vi "G#Object_UnregisterObject.vi"(0 "reference in":refnum<class "G#Object.lvclass">, 1 "object information":T1, 2 "object killed":bool, 3 "forced destroy":bool, 5 "error in (no error)":errorcluster) -> (14 "reference out":refnum<class "G#Object.lvclass">, 19 "error out":errorcluster)   [LabVIEW 2020, in "G#Object.lvclass"]
doc: "Unregisters the object from the G# object lists. It also sends an event to the debugger and desktop trace."
uses:
  <vilib>/addons/_AddQ/G#Object/G#Object.lvclass
  <vilib>/addons/_AddQ/G#Object/utils/G#Object_ObjectInfoType.ctl
  <vilib>/addons/_AddQ/G#Object/utils/G#Object_CreateMethod.ctl
  <vilib>/addons/_AddQ/G#Object/G#Object.lvclass/G#Object.ctl
  <vilib>/addons/_AddQ/G#Object/utils/G#Object_EventType.ctl
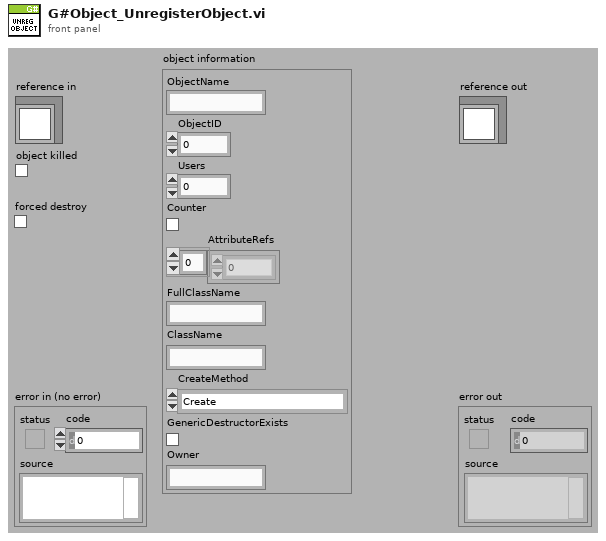
[diagram p1: front panel]
types:
  T1 = typedef "G#Object.lvclass/G#Object_ObjectInfoType.ctl" = cluster{"ObjectName":string, "ObjectID":u32, "Users":i32, "Counter":bool, "AttributeRefs":u32[], "FullClassName":string, "ClassName":string, "CreateMethod":T2, "GenericDestructorExists":bool, "Owner":string}
  T2 = typedef "G#Object.lvclass/G#Object_CreateMethod.ctl" = enum16{"Create", "Create or look up existing", "Look up existing"}
  T3 = typedef "G#Object.lvclass/G#Object_EventType.ctl" = enum16{"Created new", "Looked up existing", "Deleted", "Forced delete", "Not deleted", "Garbage collected", "Cleared", "User", "Error", "External create object", "External create class attributes", "Created class attributes", "Run constructor", "Run constructor done", "Run open method", "Run open method done"}
  T4 = cluster{"full class name (\"\")":string, "Ref":refnum<class "G#Object.lvclass">}
  T5 = cluster{"full class name (\"\")":string, "Ref":refnum<class "G#Object.lvclass">}[]
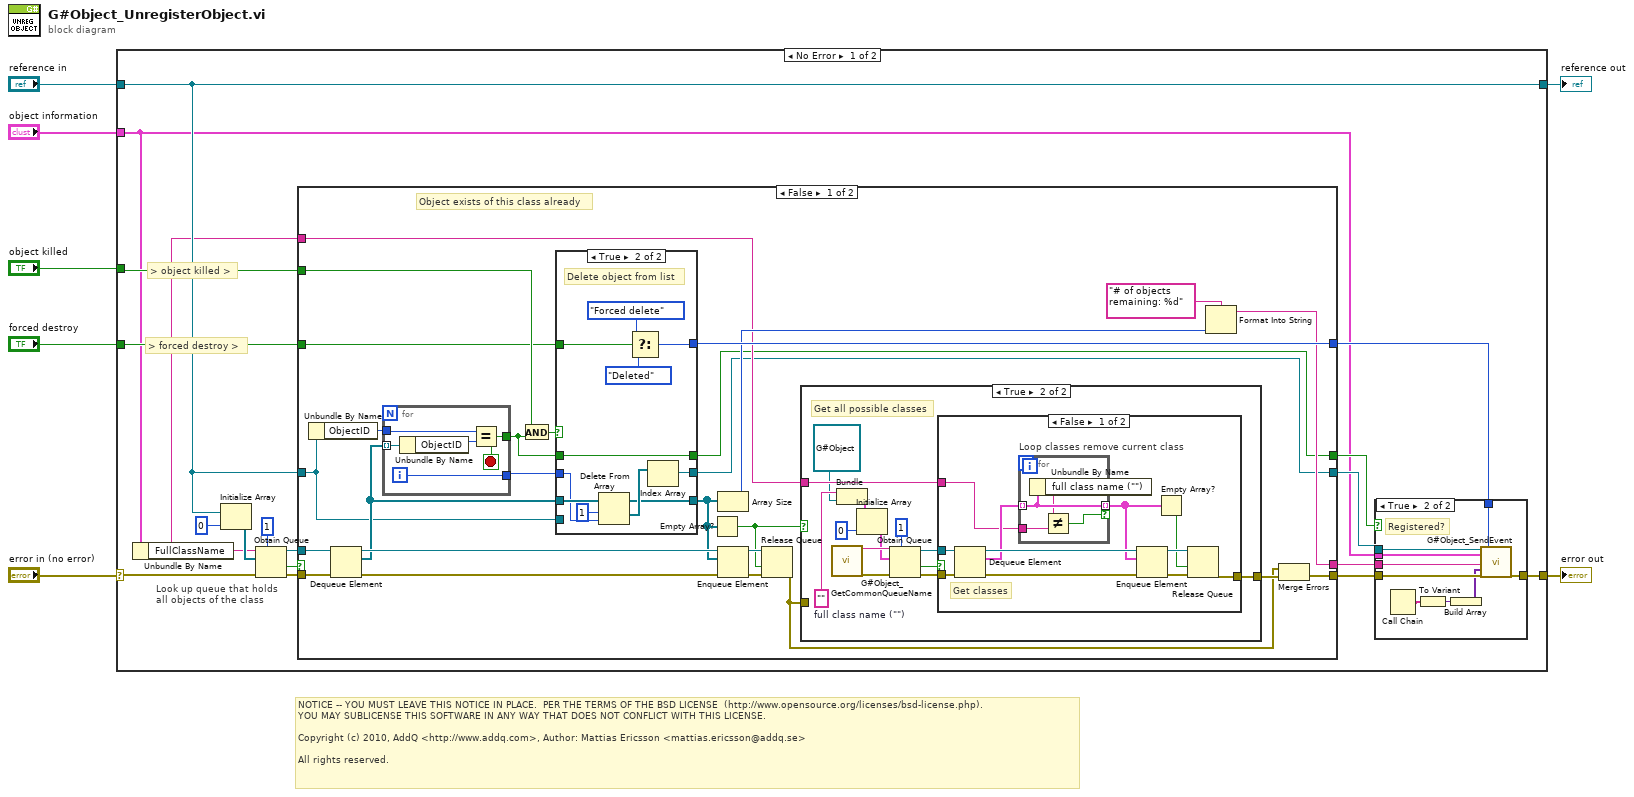
[diagram p0: block diagram]
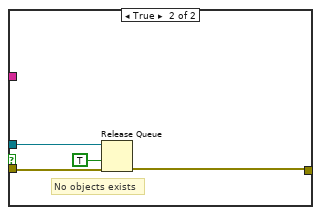
[diagram p4: hidden frame]
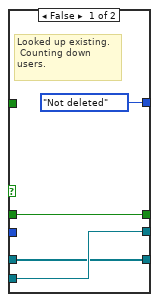
[diagram p5: hidden frame]
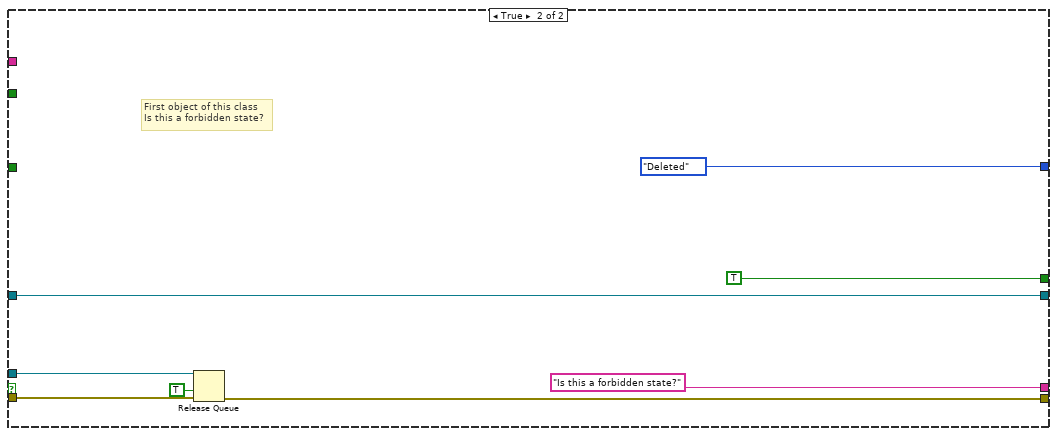
[diagram p6: hidden frame]
diagram:
  # "NOTICE -- YOU MUST LEAVE THIS NOTICE IN PLACE.  PER THE TERMS OF THE BSD LICENSE  (http://www.opensource.org/licenses/bsd-license.php).\nYOU MAY SUBLICENSE THIS SOFTWARE IN ANY WAY THAT DOES NOT CONFLICT WITH THIS LICENSE.\n\nCopyright (c) 2010, AddQ <http://www.addq.com>, Author: Mattias Ericsson <mattias.ericsson@addq.se>\n\nAll rights reserved."
  n1 = case shown="No Error" "error in (no error)" {
    selector: "error in (no error)" -> [w15 w123]
    tunnel: [w16 w123] -> w6
    tunnel: [w14 w122] -> w4
    tunnel: "reference in" -> [w14 w122]
    tunnel: "object killed" -> [w18 _]
    tunnel: "forced destroy" -> [w17 _]
    tunnel: "object information" -> [w9 _]
    frame No Error {
      # "> object killed >"
      # "> forced destroy >"
      # "Look up queue that holds\nall objects of the class"
      n2 = Unbundle By Name(w9) -> ("FullClassName"=w8:string)
      n3 = Initialize Array(w14, 0 ("dimension size")) -> (w12:refnum<class "G#Object.lvclass">[])
      n4 = Obtain Queue(max queue size (-1, unlimited)=1, name (unnamed)=w8, element data type=w12, error in (no error)=w15) -> (queue out=w22:refnum<queue>, created new?=w23:bool, error out=w24:errorcluster)  [unwired: 1 in]
      n5 = case shown="False" w23 {
        tunnel: w24 -> [w61 w121]
        tunnel: w22 -> [w60 w119]
        tunnel: [w37 w120] -> w21
        tunnel: w14 -> [w48 w118]
        tunnel: w18 -> [w53 _]
        tunnel: w17 -> [w52 _]
        tunnel: [w40 w118] -> w10
        tunnel: [w50 G#Object_EventType."Deleted" ("G#Event")] -> w20
        tunnel: [w45 "Is this a forbidden state?"] -> w19
        tunnel: [w41 TRUE] -> w11
        tunnel: w8 -> [w42 _]
        frame False {
          # "Object exists of this class already"
          n6 = Unbundle By Name(w48) -> ("ObjectID"=w49:u32)
          n7 = Dequeue Element(queue=w60, error in (no error)=w61) -> (queue out=w59:refnum<queue>, element=w55:refnum<class "G#Object.lvclass">[], error out=w58:errorcluster)  [unwired: 1 in, 1 out]
          n8 = for {
            tunnel: w55 -> [w113] mode=indexing
            tunnel: w49 -> [w111]
            tunnel: [w110] -> w51
            tunnel: [w109] -> w44
            i -> [w110]
            stop <- w109 stop-if-true
            n9 = Unbundle By Name(w113) -> ("ObjectID"=w112:u32)
            n10 = Equal?(x=w111, y=w112) -> (x = y?=w109:bool)
          }
          n11 = And(x=w53, y=w44) -> (x .and. y?=w54:bool)
          n12 = case shown="True" w54 {
            tunnel: w55 -> [w95 w108]
            tunnel: [w95 w99] -> w43
            tunnel: w52 -> [_ w106]
            tunnel: [w96 w101] -> w40
            tunnel: w51 -> [_ w102]
            tunnel: [G#Object_EventType."Not deleted" ("G#Event") w103] -> w50
            tunnel: w48 -> [w96 _]
            tunnel: w44 -> [w94 w98]
            tunnel: [w94 w98] -> w41
            frame False {
              # "Looked up existing.\n Counting down\nusers."
            }
            frame True {
              # "Delete object from list"
              n13 = Delete From Array(array=w108, length=1, index=w102) -> (deleted portion=w100:refnum<class "G#Object.lvclass">[], array with subset deleted=w99:refnum<class "G#Object.lvclass">[])
              n14 = Select(t=G#Object_EventType."Forced delete" ("G#Event"), s=w106, f=G#Object_EventType."Deleted" ("G#Event")) -> (s? t:f=w103:T3)
              n15 = Index Array(array=w100) -> (element=w101:refnum<class "G#Object.lvclass">)  [unwired: 1 in]
            }
          }
          n16 = Empty Array?(array=w43) -> (empty?=w39:bool)
          n17 = Array Size(array=w43) -> (size(s)=w46:i32)
          n18 = Enqueue Element(queue=w59, element=w43, error in (no error)=w58) -> (queue out=w56:refnum<queue>, error out=w57:errorcluster)  [unwired: 1 in, 1 out]
          n19 = Release Queue(queue=w56, force destroy? (F)=w39, error in (no error)=w57) -> (error out=w36:errorcluster)  [unwired: 2 out]
          n20 = case shown="True" w39 {
            tunnel: [_ w69] -> w38
            tunnel: w42 -> [_ w63]
            tunnel: w36 -> [_ _]
            frame False {
              # "Still existing classes"
            }
            frame True {
              w64 = ""  # full class name ("")
              # "Get all possible classes"
              n21 = call <vilib>:"G#Object_GetCommonQueueName.vi"() -> ("queue name"=w66:string, "error out"=w67:errorcluster)  [unwired: 18 in]
              n22 = Bundle("full class name (\"\")"=w64, "Ref"=refnum<class "G#Object.lvclass"> refnum) -> (w68:T4)  [unwired: 1 in]
              n23 = Initialize Array(w68, 0 ("dimension size")) -> (w65:T5)
              n24 = Obtain Queue(max queue size (-1, unlimited)=1, name (unnamed)=w66, element data type=w65, error in (no error)=w67) -> (queue out=w72:refnum<queue>, created new?=w74:bool, error out=w73:errorcluster)  [unwired: 1 in]
              n25 = case shown="False" w74 {
                tunnel: w73 -> [w79 w91]
                tunnel: w72 -> [w81 w92]
                tunnel: [w85 w93] -> w69
                tunnel: w63 -> [w77 _]
                frame False {
                  # "Get classes"
                  n26 = Dequeue Element(queue=w81, error in (no error)=w79) -> (queue out=w80:refnum<queue>, element=w78:T5, error out=w75:errorcluster)  [unwired: 1 in, 1 out]
                  n27 = for "Loop classes remove current class" {
                    tunnel: w78 -> [w89] mode=indexing
                    tunnel: w77 -> [w87]
                    tunnel: [w89] -> w76 mode=indexing if=w86
                    n28 = Unbundle By Name(w89) -> ("full class name (\"\")"=w88:string)
                    n29 = Not Equal?(x=w88, y=w87) -> (x != y?=w86:bool)
                  }
                  n30 = Enqueue Element(queue=w80, element=w76, error in (no error)=w75) -> (queue out=w83:refnum<queue>, error out=w84:errorcluster)  [unwired: 1 in, 1 out]
                  n31 = Empty Array?(array=w76) -> (empty?=w82:bool)
                  n32 = Release Queue(queue=w83, force destroy? (F)=w82, error in (no error)=w84) -> (error out=w85:errorcluster)  [unwired: 2 out]
                }
                frame True {
                  # "No objects exists"
                  n33 = Release Queue(queue=w92, force destroy? (F)=TRUE, error in (no error)=w91) -> (error out=w93:errorcluster)  [unwired: 2 out]
                }
              }
            }
          }
          n34 = Format Into String(format string="# of objects remaining: %d", w46) -> (resulting string=w45:string)  [unwired: 2 in, 1 out]
          n35 = Merge Errors(w36, w38) -> (w37:errorcluster)
        }
        frame True {
          # "First object of this class\nIs this a forbidden state?"
          n36 = Release Queue(queue=w119, force destroy? (F)=TRUE, error in (no error)=w121) -> (error out=w120:errorcluster)  [unwired: 2 out]
        }
      }
      n37 = case shown="True" w11 {
        tunnel: w21 -> [w26 w35]
        tunnel: w20 -> [_ w34]
        tunnel: w19 -> [_ w33]
        tunnel: [w26 w32] -> w16
        tunnel: w9 -> [_ w31]
        tunnel: w10 -> [_ w30]
        frame False {
        }
        frame True {
          # "Registered?"
          n38 = Call Chain() -> (call chain=w29:string[])
          n39 = To Variant(anything=w29) -> (Variant=w28:variant)
          n40 = Build Array(w28) -> (w27:variant[])
          n41 = call <vilib>:"G#Object_SendEvent.vi"("reference in"=w30, "object info extended"=w31, "comment"=w33, "parameters"=w27, "error in (no error)"=w35, "G# event type"=w34) -> ("error out"=w32:errorcluster)  [unwired: 13 in]
        }
      }
    }
    frame Error {
    }
  }
  "error out" <- w6
  "reference out" <- w4
